vi "Expt10a_MT BCH Encode-Decode_Student_lab.vi"() -> ()   [LabVIEW 2020]
doc: "This example demonstrates BCH Channel coding and decoding."
uses:
  <vilib>/addons/Modulation/Digital/General/MT Generate Bits (Galois, PN Order).vi
  <vilib>/addons/Modulation/niDMT.lvlib
panel:
  out "Bit Error Rate (no coding)":dbl format="%.4f"
  out "Error Out":errorcluster
  out "Encoded Bit Count":i32
  in  "n,k,t":string(combo)="127,85,6"
  out "Noise":i8[](array[numeric])
  out "Bit Error Rate":dbl
  in  "Noise (bit flip probability)":dbl=0.01 format="%.6g"
  out "Message Bits":i8[](array[numeric])
  out "Encoded Bits":i8[](array[numeric])
  out "Decoded Bits":i8[](array[numeric])
  in  "Message Bits":i32=1000
  # "BCH Code / Decode Programming Example"
  # "code word length (n),\ndata word length (k),\nmax errors corrected (t)"
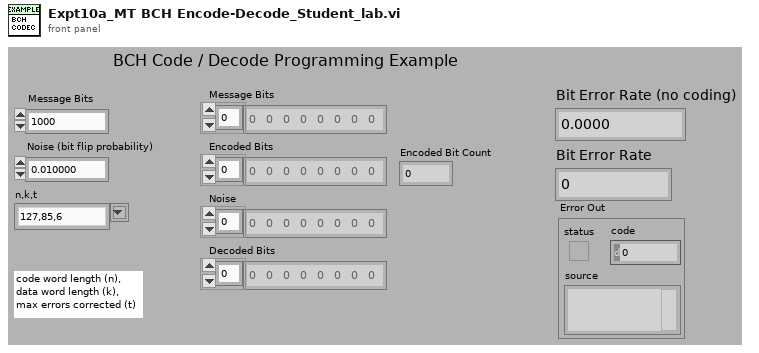
[diagram p1: front panel]
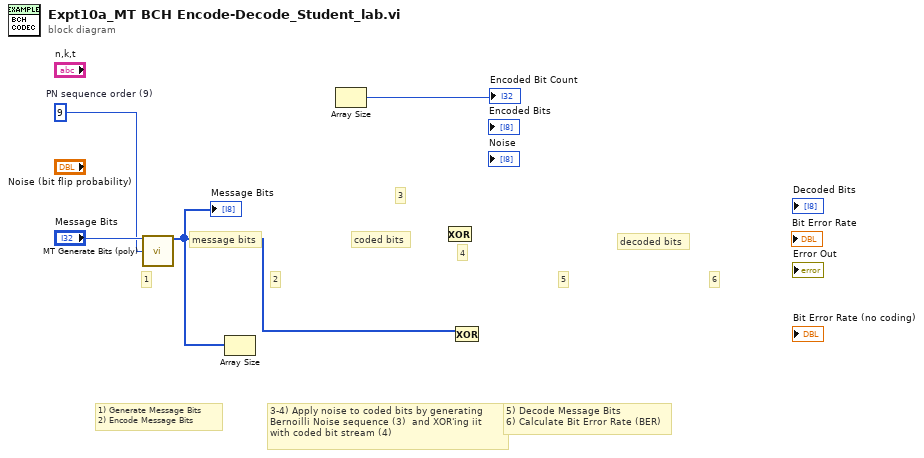
[diagram p0: block diagram]
diagram:
  w1 = 9  # PN sequence order (9)
  # "decoded bits"
  # "message bits"
  # "coded bits"
  # "6"
  # "5"
  # "4"
  # "3"
  # "2"
  # "1"
  # "5) Decode Message Bits\n6) Calculate Bit Error Rate (BER)"
  # "1) Generate Message Bits\n2) Encode Message Bits"
  # "3-4) Apply noise to coded bits by generating \nBernoilli Noise sequence (3)  and XOR'ing iit \nwith coded bit stream (4)"
  n1 = call-poly <vilib>:"MT Generate Bits (poly).vi"("total bits (128)"="Message Bits", "PN sequence order (9)"=w1) -> ("output bit stream"=w2:i8[])  [unwired: 11 in, 2 out]
  "Message Bits" <- w2
  n2 = Array Size(array=w2) -> ()  [unwired: 1 out]
  n3 = Array Size() -> (size(s)=→"Encoded Bit Count":i32)  [unwired: 1 in]
  n4 = Exclusive Or() -> ()  [unwired: 2 in, 1 out]
  n5 = Exclusive Or(2:w2) -> ()  [unwired: 1 in, 1 out]
